vi "Phase_estimation.vi"() -> ()   [LabVIEW 2022 SP3]
uses:
  <vilib>/platform/TimedLoop/XDataNode/XDataNode.xnode
  <vilib>/Platform/TimedLoop/XDataNode/timing_clust.ctl
  <vilib>/Platform/TimedLoop/XDataNode/XDNodeRunTimeDep.lvlib
  <vilib>/Platform/TimedLoop/XDataNode/wakeup.ctl
  <vilib>/Platform/TimedLoop/XDataNode/nitl_modes.ctl
  <vilib>/rvi/DataTransferAndStorage/Container/XNode/niFpgaContainer.xnode
  <vilib>/rvi/FIFO/Fifo_Resource/niFpgaFifoEmulationRefIn.vi
  <vilib>/rvi/Memory/Memory_Emulation/niFpgaMemoryEmulationRefIn.vi
  <vilib>/eio/EIONode/EIONode.xnode
  <vilib>/rvi/eio/common/nirviEmuTemplateMethod_errors.vi
  <vilib>/rvi/FXPMathLib/FxpConvert/XNode/nifxpmath_Convert.xnode
  <vilib>/rvi/FXPMathLib/FxpConvert/subVIs/nifxpmath_Convert_SimConfig.ctl
  <vilib>/fxp/LVFixedPointOverflowPolicyTypeDef.ctl
  <vilib>/fxp/LVFixedPointQuantizationPolicyTypeDef.ctl
  <vilib>/rvi/FXPMathLib/FxpConvert/simVIs/DllFxpConvertTemp_sub.vi
  <vilib>/rvi/FXPMathLib/FxpSub/XNode/nifxpmath_Sub.xnode
  <vilib>/rvi/FXPMathLib/FxpSinAndCos/XNode/nifxpmath_SinAndCos.xnode
  <vilib>/rvi/FXPMathLib/FxpMul/XNode/nifxpmath_Multiplier.xnode
  <vilib>/rvi/FXPMathLib/basic elements/DSP48E/XNode/niFpgaDsp48e.xnode
  <vilib>/rvi/FXPMathLib/basic elements/DSP48E/subVIs/niFpgaDsp48eAutoresetState.ctl
  <vilib>/rvi/FXPMathLib/basic elements/DSP48E/subVIs/niFpgaDsp48eSelectMaskState.ctl
  <vilib>/rvi/FXPMathLib/basic elements/DSP48E/subVIs/niFpgaDsp48eSelectPatternState.ctl
  <vilib>/rvi/FXPMathLib/basic elements/DSP48E/subVIs/niFpgaDsp48eLogicUnitModeState.ctl
  <vilib>/rvi/FXPMathLib/basic elements/DSP48E/subVIs/niFpgaDsp48eUseMultiplierState.ctl
  <vilib>/rvi/FXPMathLib/basic elements/DSP48E/subVIs/niFpgaDsp48eAlumodeOpmodeCarryinselState.ctl
  <vilib>/rvi/FXPMathLib/basic elements/DSP48E/subVIs/niFpgaDsp48eType.ctl
  <vilib>/rvi/FXPMathLib/basic elements/DSP48E/simVIs/niFpgaDsp48eSimulationState.ctl
  <vilib>/rvi/FXPMathLib/basic elements/DSP48E/simVIs/niFpgaDsp48eResets.ctl
  <vilib>/rvi/FXPMathLib/basic elements/DSP48E/simVIs/niFpgaDsp48eEnables.ctl
  <vilib>/rvi/FXPMathLib/basic elements/DSP48E/simVIs/niFpgaDsp48eRegisters.ctl
  <vilib>/rvi/FXPMathLib/basic elements/DSP48E/simVIs/niFpgaDsp48eSimMultiplier.vi
  <vilib>/rvi/FXPMathLib/basic elements/DSP48E/simVIs/niFpgaDsp48eSimArithmetic.vi
  <vilib>/rvi/FXPMathLib/basic elements/DSP48E/simVIs/niFpgaDsp48eSimPatternDetect.vi
  <vilib>/rvi/FXPMathLib/basic elements/DSP48E/simVIs/niFpgaDsp48eSimP.vi
  <vilib>/rvi/FXPMathLib/basic elements/DSP48E/simVIs/niFpgaDsp48eSimUpdateState.vi
  <vilib>/rvi/FXPMathLib/basic elements/DSP48E/simVIs/niFpgaDsp48eCheckMode.vi
  <vilib>/rvi/FXPMathLib/basic elements/DSP48E/simVIs/niFpgaDsp48eReportInvalidMode.vi
  <vilib>/rvi/FXPMathLib/sim/FxpSim.dll
  <vilib>/rvi/FXPMathLib/FxpSinAndCos/simVIs/DllFxpSinAndCosTemp_sub.vi
  <vilib>/rvi/FXPMathLib/FxpSinAndCos/subVIs/nifxpmath_SinAndCos_SimConfig.ctl
panel:
  in  "Generate Steps?":bool
  in  "White Noise\nAmplitude":u16=32768 caption="amplitude"
  in  "Add White\nNoise?":bool
  in  "Memory Debug\nMode":bool
  out "Data 2":fxp<+/-,18,-4>
  out "Data":fxp<+/-,18,-4>
  in  "Address":u32
  in  "Input? AI : Direct":bool
  out "Sgi":fxp<+/-,48,5>
  out "Sgphi":fxp<+/-,48,5>
  out "Phi":fxp<+/-,48,5>
  out "Weights Loaded":bool
  in  "psi_true":fxp<+/-,48,5>
  in  "DMA FIFO\nOutput Resolution":u32
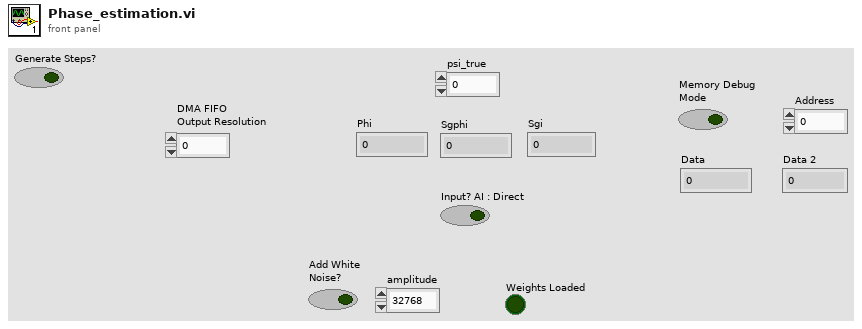
[diagram p1: front panel]
types:
  T1 = typedef "XDNodeRunTimeDep.lvlib/timing_clust.ctl" = cluster{"Expected End [f-1]":u64, "Actual End [f-1]":u64, "Finished Late? [f-1]":bool, "Expected End [i-1]":u64, "Actual End [i-1]":u64, "Finished Late? [i-1]":bool, "Expected Start [i]":u64, "Actual Start [i]":u64, "Expected Start [f]":u64, "Actual Start [f]":u64, "Source Name":string, "Structure Name":string, "Period":i64, "Deadline":i64, "Offset":i64, "Start":i64, "Priority":i32, "Timeout":i32, "Mode":T2, "Wakeup Reason":T3, "Error":errorcluster, "Source Type":string, "Secondary Source Type":string, "Global End Time":u64, "Global Start Time":u64, "Frame Duration":u64, "Iteration Duration":u64, "Assigned CPU":i32, "I/O Scan Engine Mode":u32}
  T2 = typedef "XDNodeRunTimeDep.lvlib/nitl_modes.ctl" = enum32{"No Change", "Process missed periods, maintain original phase", "Discard missed periods, maintain original phase", "Process missed periods, ignore original phase", "Discard missed periods, ignore original phase"}
  T3 = typedef "XDNodeRunTimeDep.lvlib/wakeup.ctl" = enum32{"Normal", "Aborted", "Asynchronous wakeup", "Timing source error", "Timed loop error", "Timeout"}
  T4 = typedef "niFpgaDsp48eRegisters.ctl" = cluster{"a register 1":fxp<+/-,30,30>, "a register 2":fxp<+/-,30,30>, "b register 1":fxp<+/-,18,18>, "b register 2":fxp<+/-,18,18>, "c register":fxp<+/-,48,48>, "d register":fxp<+/-,25,25>, "ad register":fxp<+/-,27,27>, "m register":fxp<+/-,45,45>, "opmode register":fxp<+,7,7>, "alumode register":fxp<+,4,4>, "carryinsel register":fxp<+,3,3>, "inmode register":fxp<+,5,5>, "carryin register":bool, "multcarryin register":bool, "p registers":fxp<+/-,48,48>, "carryout register":fxp<+,4,4>, "carrycascout register":bool, "multsignout register":bool, "patterndetect register":bool, "patternbdetect register":bool, "patterndetect register 2":bool, "patternbdetect register 2":bool}
  T5 = typedef "niFpgaDsp48eEnables.ctl" = cluster{"cea1":bool, "cea2":bool, "cead":bool, "cealumode":bool, "ceb1":bool, "ceb2":bool, "cec":bool, "cecarryin":bool, "cectrl":bool, "ced":bool, "ceinmode":bool, "cem":bool, "cemultcarryin":bool, "cep":bool}
  T6 = typedef "niFpgaDsp48eResets.ctl" = cluster{"rsta":bool, "rstallcarryin":bool, "rstalumode":bool, "rstb":bool, "rstc":bool, "rstctrl":bool, "rstd":bool, "rstinmode":bool, "rstm":bool, "rstp":bool}
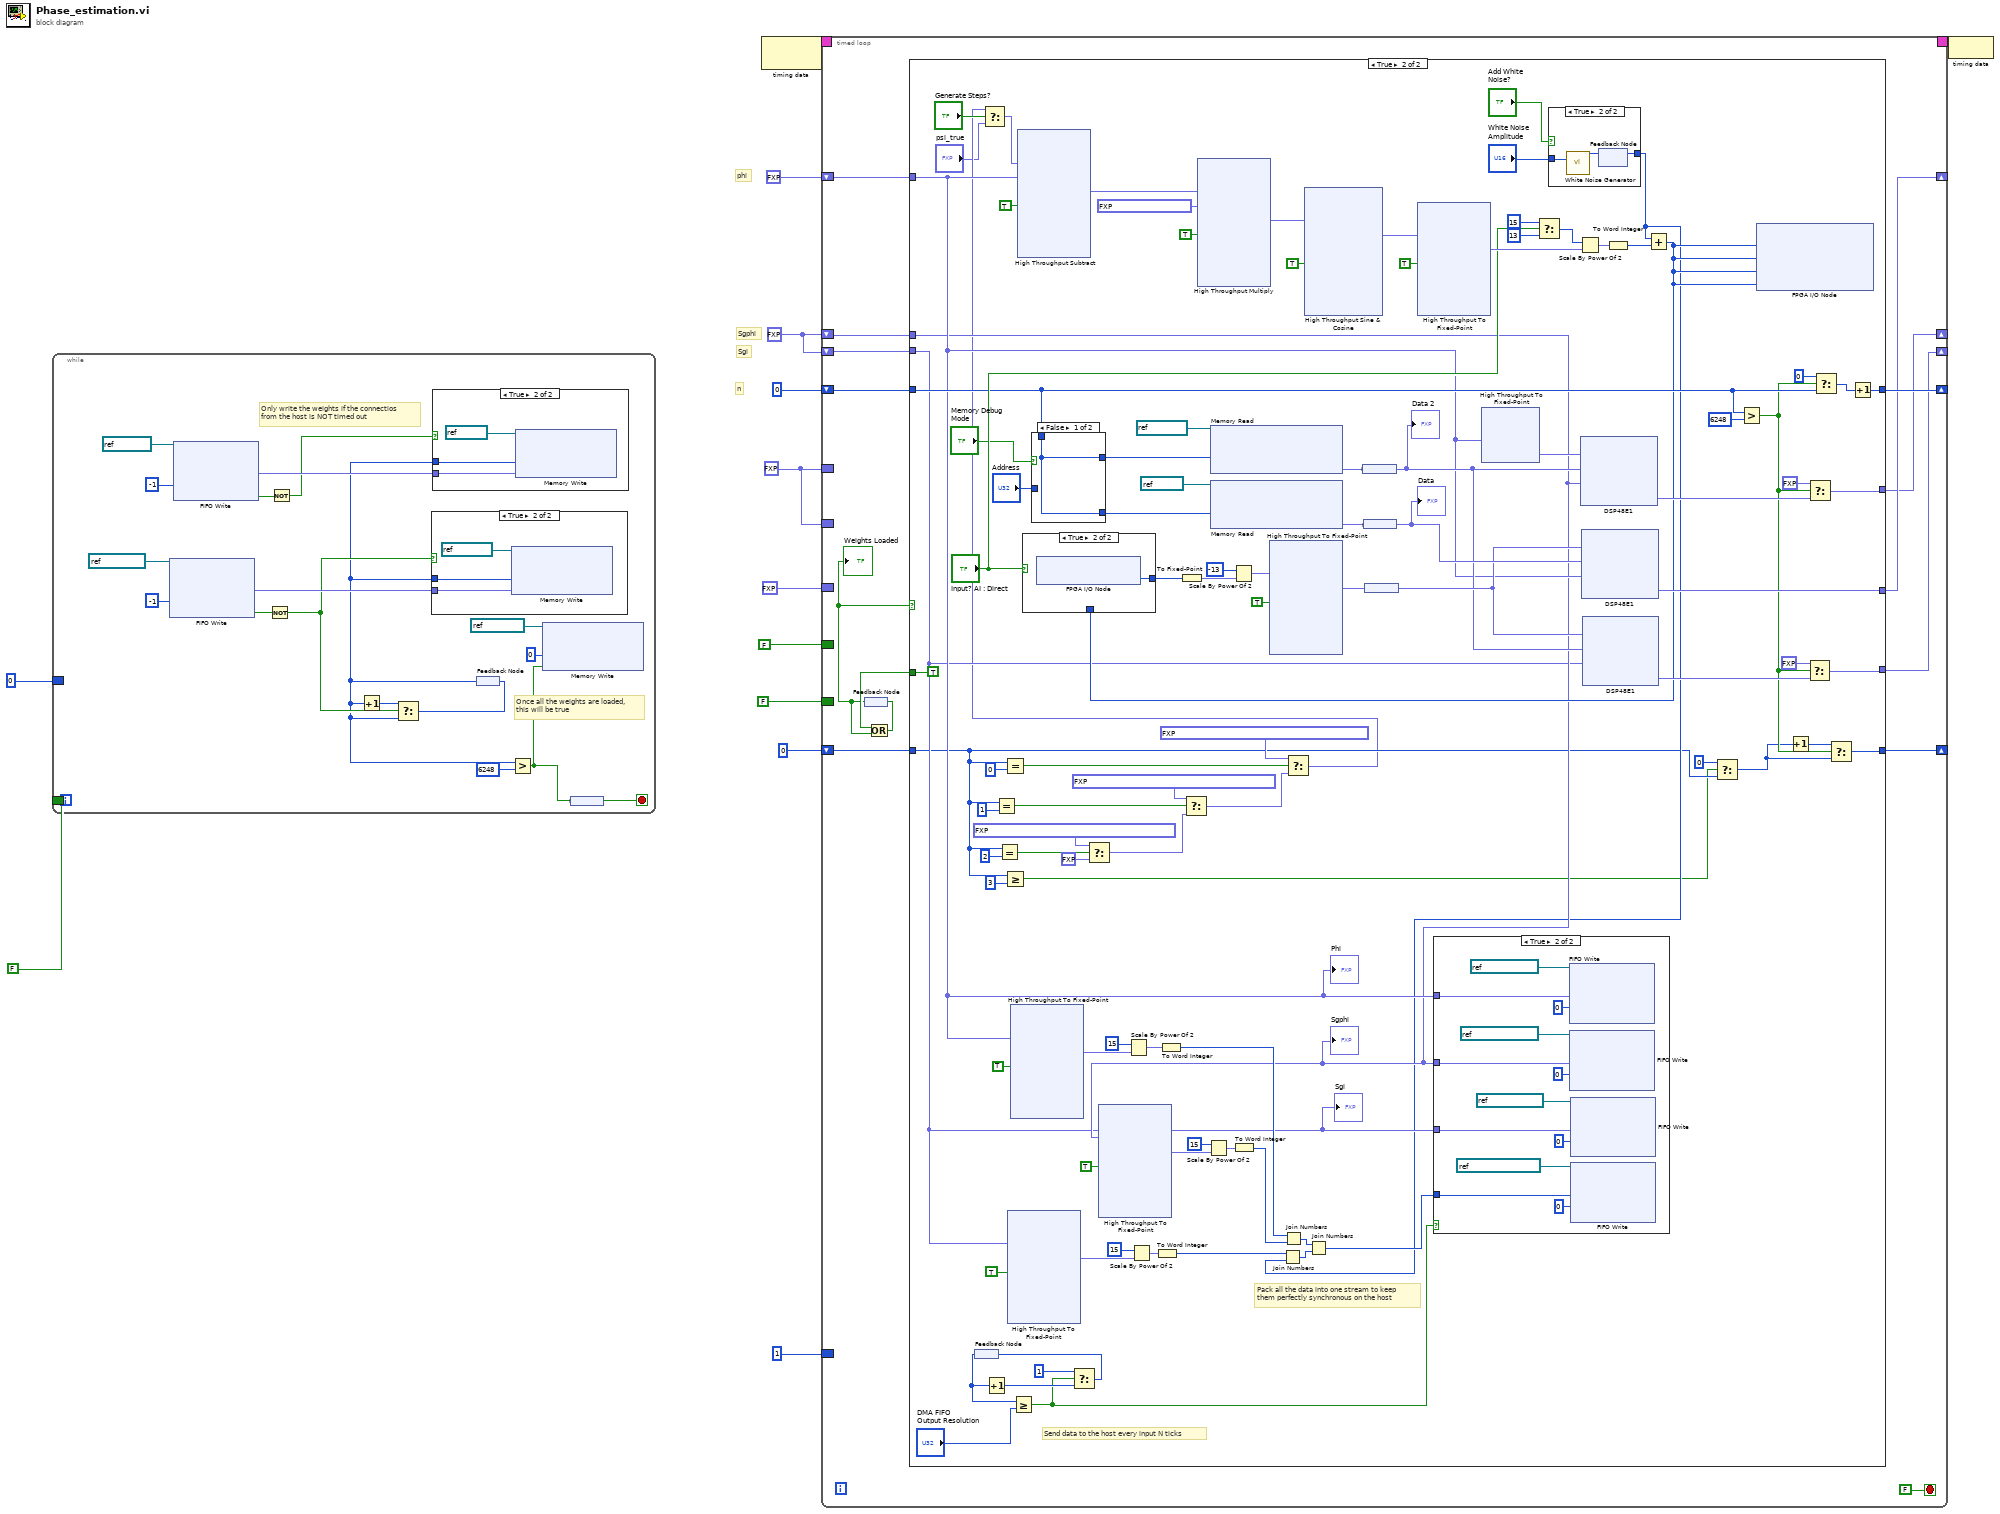
[diagram p0: block diagram]
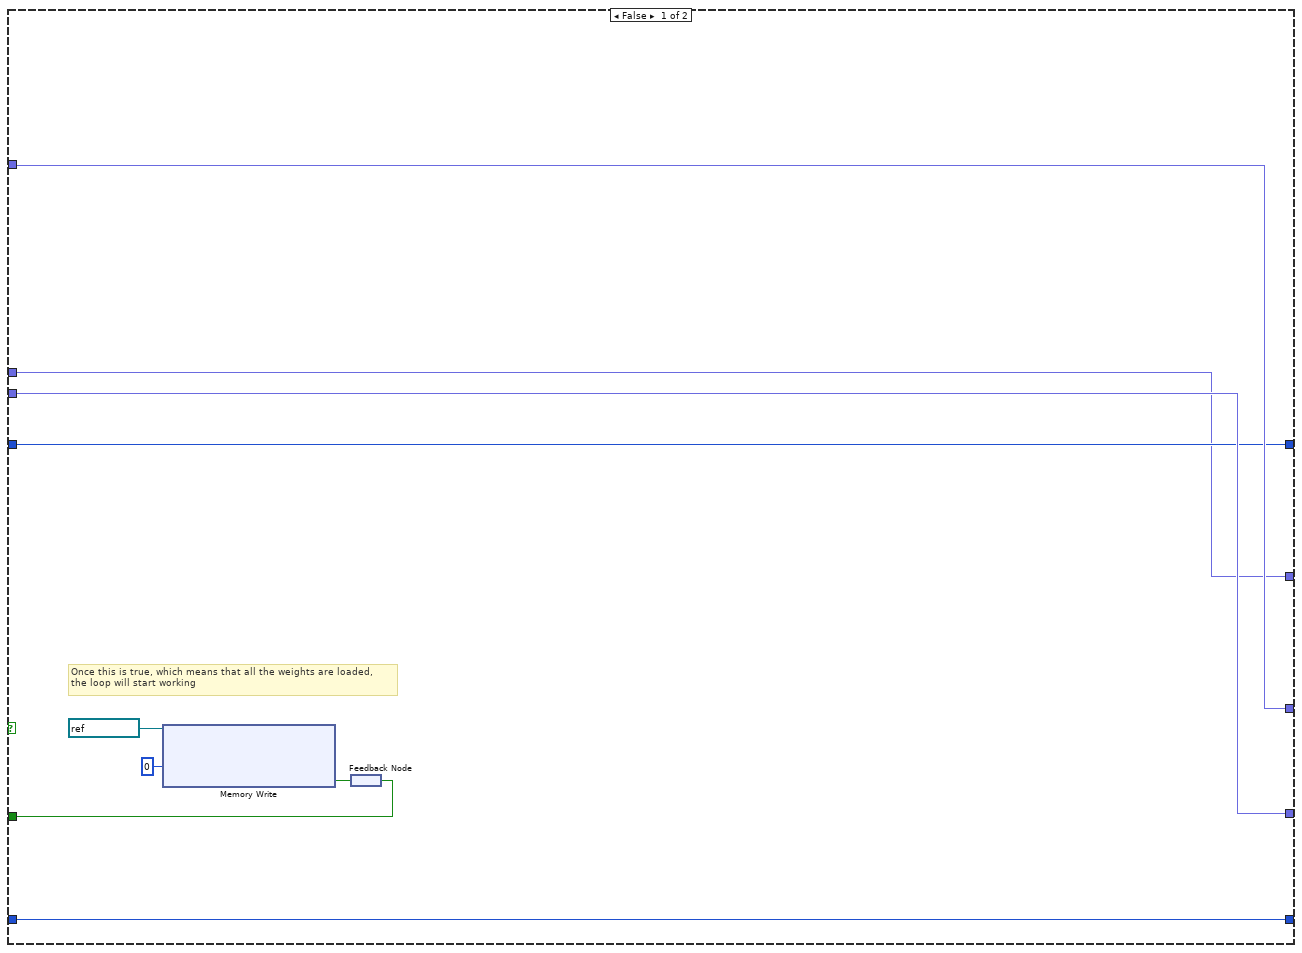
[diagram p4: hidden frame]
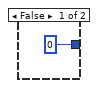
[diagram p5: hidden frame]
diagram:
  w5 = fxp<+/-,18,-4> 0.0 ("Data")
  w6 = fxp<+/-,48,5> 0.0 ("Element")
  # "n"
  # "Sgi"
  # "Sgphi"
  # "phi"
  n1 = while {
    border: u32 0 ("Element") -> [_]
    border: FALSE -> [_]
    stop <- w17 stop-if-true
    # "Once all the weights are loaded,\nthis will be true"
    # "Only write the weights if the connectios\nfrom the host is NOT timed out"
    n2 = xnode ("FIFO Write")("Timeout"=-1, "FIFO In"=refnum<k21> "FIFO_gdt") -> ("Element"=w31:fxp<+/-,18,-4>, "Timed Out?"=w24:bool)  [unwired: 1 out]
    n3 = xnode ("FIFO Write")("Timeout"=-1, "FIFO In"=refnum<k21> "FIFO_h") -> ("Element"=w30:fxp<+/-,18,-4>, "Timed Out?"=w25:bool)  [unwired: 1 out]
    n4 = Not(x=w24) -> (.not. x?=w21:bool)
    n5 = Not(x=w25) -> (.not. x?=w23:bool)
    n6 = feedback #1() -> (w19:u32)
    n7 = Increment(x=w19) -> (x+1=w20:u32)
    n8 = Select(t=w20, s=w21, f=w19) -> (s? t:f=w18:u32)
    n9 = case shown="True" w21 {
      tunnel: w31 -> [_ w36]
      tunnel: w19 -> [_ w35]
      frame False {
      }
      frame True {
        n10 = xnode ("Memory Write")("Address"=w35, "Data"=w36, "Memory In"=refnum<k21> "gdtLUT") -> ()  [unwired: 1 out]
      }
    }
    n11 = case shown="True" w23 {
      tunnel: w30 -> [_ w33]
      tunnel: w19 -> [_ w32]
      frame False {
      }
      frame True {
        n12 = xnode ("Memory Write")("Address"=w32, "Data"=w33, "Memory In"=refnum<k21> "hLUT") -> ()  [unwired: 1 out]
      }
    }
    n13 = feedback-in #1(w18) -> ()
    n14 = Greater?(x=w19, y=u32 6248) -> (0:w15:bool)
    n15 = xnode ("Memory Write")("Address"=u32 0, "Data"=w15, "Memory In"=refnum<k21> "Boolean") -> ()  [unwired: 1 out]
    n16 = feedback #2() -> (w17:bool)
    n17 = feedback-in #2(w15) -> ()
  }
  n18 = node-c288() -> (w13:T1)  [unwired: 1 in]
  n19 = timed-loop {
    timing: w13 -> [_]
    timing-out: [_] -> w12
    border: u32 1 ("Timeout") -> [_]
    shift-right: [w48] -> _
    shift-left: fxp<+/-,48,5> 0.0 ("Element") -> [w44]
    shift-right: [w43] -> _
    shift-left: w6 -> [w47]
    shift-right: [w46] -> _
    shift-left: w6 -> [w45]
    shift-right: [w50] -> _
    shift-left: u32 0 ("Element") -> [w49]
    border: FALSE -> [_]
    border: w5 -> [_]
    border: w5 -> [_]
    border: fxp<+/-,25,4> 0.0 ("Data") -> [_]
    border: FALSE -> [_]
    shift-right: [w39] -> _
    shift-left: u32 0 ("Element") -> [w38]
    stop <- FALSE stop-if-true
    n20 = feedback #3() -> (w40:bool)
    "Weights Loaded" <- w40
    n21 = case shown="True" w40 {
      tunnel: [w58 w147] -> w50
      tunnel: w49 -> [w58 w119]
      tunnel: [w60 w95] -> w48
      tunnel: w47 -> [w57 w88]
      tunnel: [w57 w136] -> w43
      tunnel: [w59 w93] -> w46
      tunnel: w45 -> [w59 w87]
      tunnel: w44 -> [w60 w111]
      tunnel: [w53 TRUE ("Data")] -> w41
      tunnel: [w52 w83] -> w39
      tunnel: w38 -> [w52 w68]
      frame False {
        # "Once this is true, which means that all the weights are loaded,\nthe loop will start working"
        n22 = xnode ("Memory Write")("Address"=u32 0, "Memory In"=refnum<k21> "Boolean") -> ("Data"=w54:bool)  [unwired: 1 out]
        n23 = feedback #4() -> (w53:bool)
        n24 = feedback-in #4(w54) -> ()
      }
      frame True {
        # "Pack all the data into one stream to keep\nthem perfectly synchronous on the host"
        # "Send data to the host every input N ticks"
        n25 = feedback #5() -> (w161:u32)
        n26 = Increment(x=w161) -> (x+1=w160:u32)
        n27 = Equal?(x=w68, y=u32 1) -> (x = y?=w78:bool)
        n28 = Equal?(x=w68, y=u32 2) -> (x = y?=w75:bool)
        n29 = Equal?(x=w68, y=u32 0) -> (x = y?=w81:bool)
        n30 = Greater Or Equal?(x=w68, y=u32 3) -> (x >= y?=w65:bool)
        n31 = xnode "High Throughput To Fixed-Point"("x"=w87, "input valid"=TRUE) -> ("y"=w110:fxp<+/-,64,16>)  [unwired: 1 in, 2 out]
        n32 = xnode "High Throughput To Fixed-Point"("x"=w111, "input valid"=TRUE) -> ("y"=w112:fxp<+/-,64,16>)  [unwired: 1 in, 2 out]
        n33 = Greater Or Equal?(x=w161, y="DMA FIFO\nOutput Resolution") -> (x >= y?=w96:bool)
        n34 = case shown="False" "Memory Debug\nMode" {
          tunnel: [w238 w239] -> w120
          tunnel: w119 -> [w238 _]
          tunnel: [w238 w239] -> w118
          tunnel: "Address" -> [_ w239]
          frame False {
          }
          frame True {
          }
        }
        n35 = Select(t=u32 1, s=w96, f=w160) -> (s? t:f=w158:u32)
        n36 = feedback-in #5(w158) -> ()
        n37 = Select(t=fxp<+/-,48,5> 0.20000000000004547 ("Element"), s=w75, f=fxp<+/-,48,5> 0.0) -> (s? t:f=w70:fxp<+/-,48,5>)
        n38 = xnode "High Throughput To Fixed-Point"("x"=w88, "input valid"=TRUE) -> ("y"=w106:fxp<+/-,64,16>)  [unwired: 1 in, 2 out]
        n39 = Scale By Power Of 2(n=i16 15, x=w112) -> (x*2^n=w104:fxp<+/-,64,16>)
        n40 = Scale By Power Of 2(n=i16 15, x=w110) -> (x*2^n=w102:fxp<+/-,64,16>)
        n41 = To Word Integer(number=w102) -> (16bit integer=w99:i16)
        n42 = To Word Integer(number=w104) -> (16bit integer=w101:i16)
        n43 = Select(t=fxp<+/-,48,5> 0.2999999999999545 ("Element"), s=w78, f=w70) -> (s? t:f=w71:fxp<+/-,48,5>)
        n44 = Scale By Power Of 2(n=i16 15, x=w106) -> (x*2^n=w103:fxp<+/-,64,16>)
        n45 = xnode ("Memory Read")("Address"=w120, "Memory In"=refnum<k21> "gdtLUT") -> ("Data"=w130:fxp<+/-,18,-4>)  [unwired: 1 out]
        n46 = xnode ("Memory Read")("Address"=w118, "Memory In"=refnum<k21> "hLUT") -> ("Data"=w129:fxp<+/-,18,-4>)  [unwired: 1 out]
        n47 = To Word Integer(number=w103) -> (16bit integer=w100:i16)
        n48 = Join Numbers(hi=w101, lo=w100) -> ((hi.lo)=w98:u32)
        n49 = Select(t=fxp<+/-,48,5> 0.10000000000002274 ("Element"), s=w81, f=w71) -> (s? t:f=w63:fxp<+/-,48,5>)
        n50 = Select(t=w63, s="Generate Steps?", f="psi_true") -> (s? t:f=w61:fxp<+/-,48,5>)
        n51 = xnode ("High Throughput Subtract")("x"=w61, "y"=w111, "input valid"=TRUE) -> ("x-y"=w153:fxp<+/-,49,6>)  [unwired: 1 in, 2 out]
        n52 = xnode ("High Throughput Multiply")("x"=w153, "y"=fxp<+/-,22,2> 0.3183097839355469, "input valid"=TRUE) -> ("x*y"=w151:fxp<+/-,64,8>)  [unwired: 1 in, 2 out]
        n53 = xnode ("High Throughput Sine & Cosine")("x (pi)"=w151, "input valid"=TRUE) -> ("sin(x)"=w150:fxp<+/-,16,2>)  [unwired: 1 in, 3 out]
        n54 = feedback #6() -> (w121:fxp<+/-,18,-4>)
        "Data 2" <- w121
        n55 = feedback-in #6(w130) -> ()
        n56 = feedback #7() -> (w134:fxp<+/-,18,-4>)
        "Data" <- w134
        n57 = feedback-in #7(w129) -> ()
        n58 = feedback #8() -> (w133:fxp<+/-,25,4>)
        n59 = xnode "High Throughput To Fixed-Point"("x"=w150, "input valid"=TRUE) -> ("y"=w149:fxp<+/-,32,16>)  [unwired: 1 in, 2 out]
        n60 = xnode "High Throughput To Fixed-Point"("x"=w111) -> ("y"=w127:fxp<+/-,25,4>)
        n61 = Select(t=i16 15 ("n"), s="Input? AI : Direct", f=i16 13 ("n")) -> (s? t:f=w123:i16)
        n62 = case shown="True" "Add White\nNoise?" {
          tunnel: [i16 0 ("white noise out") w164] -> w85
          tunnel: "White Noise\nAmplitude" -> [_ w163]
          frame False {
          }
          frame True {
            n63 = call "White Noise Generator"("RMS"=w163) -> ("white noise out"=w165:i16)  [unwired: 13 in, 1 out]
            n64 = feedback #9() -> (w164:i16)  [unwired: 1 in]
            n65 = feedback-in #9(w165) -> ()
          }
        }
        n66 = Join Numbers(hi=w99, lo=w85) -> ((hi.lo)=w97:u32)
        n67 = Join Numbers(hi=w98, lo=w97) -> ((hi.lo)=w86:u64)
        n68 = case shown="True" w96 {
          tunnel: w111 -> [_ w537]
          tunnel: w88 -> [_ w529]
          tunnel: w87 -> [_ w528]
          tunnel: w86 -> [_ w527]
          frame False {
          }
          frame True {
            n69 = xnode ("FIFO Write")("Element"=w537, "Timeout"=0, "FIFO In"=refnum<k21> "Phi_ToHost") -> ()  [unwired: 2 out]
            n70 = xnode ("FIFO Write")("Element"=w529, "Timeout"=0, "FIFO In"=refnum<k21> "Sgphi_ToHost") -> ()  [unwired: 2 out]
            n71 = xnode ("FIFO Write")("Element"=w528, "Timeout"=0, "FIFO In"=refnum<k21> "Sgi_ToHost") -> ()  [unwired: 2 out]
            n72 = xnode ("FIFO Write")("Element"=w527, "Timeout"=0, "FIFO In"=refnum<k21> "Packed_ToHost") -> ()  [unwired: 2 out]
          }
        }
        n73 = Scale By Power Of 2(n=w123, x=w149) -> (x*2^n=w148:fxp<+/-,32,16>)
        n74 = xnode ("DSP48E1")("a"=w127, "b"=w121, "c"=w88) -> ("p"=w135:fxp<+/-,48,5>)
        n75 = xnode ("DSP48E1")("a"=w133, "b"=w134, "c"=w111) -> ("p"=w95:fxp<+/-,48,5>)
        n76 = xnode ("DSP48E1")("a"=w133, "b"=w121, "c"=w87) -> ("p"=w94:fxp<+/-,48,5>)
        n77 = To Word Integer(number=w148) -> (16bit integer=w91:i16)
        n78 = Add(x=w85, y=w91) -> (x+y=w90:i16)
        n79 = case shown="True" "Input? AI : Direct" {
          tunnel: [w240 w241] -> w126
          tunnel: w90 -> [w240 _]
          frame False {
          }
          frame True {
            n80 = xnode "FPGA I/O Node"() -> ("IO Module\\AI 1 N"=w241:i16)  [unwired: 1 in, 1 out]
          }
        }
        n81 = To Fixed-Point(number=w126) -> (fixed-point=w155:fxp<+/-,38,16>)  [unwired: 1 in]
        n82 = Scale By Power Of 2(n=i16 -13, x=w155) -> (x*2^n=w154:fxp<+/-,38,16>)
        n83 = xnode "High Throughput To Fixed-Point"("x"=w154, "input valid"=TRUE) -> ("y"=w141:fxp<+/-,25,4>)  [unwired: 1 in, 2 out]
        n84 = feedback-in #8(w141) -> ()
        n85 = Select(t=u32 0, s=w65, f=w68) -> (s? t:f=w67:u32)
        n86 = Greater?(x=w119, y=u32 6248) -> (0:w69:bool)
        n87 = xnode "FPGA I/O Node"("IO Module\\AO 1 N"=w90, "IO Module\\AO 1 N-1"=w90, "IO Module\\AO 1 N-2"=w90, "IO Module\\AO 1 N-3"=w90) -> ()  [unwired: 4 in, 4 out]
        n88 = Increment(x=w67) -> (x+1=w84:u32)
        n89 = Select(t=fxp<+/-,48,5> 0.0, s=w69, f=w94) -> (s? t:f=w93:fxp<+/-,48,5>)
        n90 = Select(t=fxp<+/-,48,5> 0.0, s=w69, f=w135) -> (s? t:f=w136:fxp<+/-,48,5>)
        n91 = Select(t=u32 0, s=w69, f=w119) -> (s? t:f=w140:u32)
        n92 = Select(t=w84, s=w69, f=w67) -> (s? t:f=w83:u32)
        n93 = Increment(x=w140) -> (x+1=w147:u32)
        "Phi" <- w111
        "Sgphi" <- w88
        "Sgi" <- w87
      }
    }
    n94 = Or(x=w41, y=w40) -> (x .or. y?=w42:bool)
    n95 = feedback-in #3(w42) -> ()
  }
  n96 = node-c288(w12) -> ()
